vi "Autonomous Independent.vi"() -> ()   [LabVIEW 2016]
doc: "This VI is called when autonomous begins, and will automatically be terminated when autonomous ends. You can carry out timed or sensor driven robot movement independently without needing to return to the caller."
uses:
  <vilib>/Rock Robotics/WPI/Relay/WPI_RelayValue.ctl
  <vilib>/Rock Robotics/WPI/Utilities/WPI_GetSetVariantRefNum.vi
  <vilib>/Rock Robotics/Network Tables/NT Write Numeric Array.vi
  <vilib>/Rock Robotics/Network Tables/NT Read String.vi
  encoder reset.vi
  Encoder Distance.vi
  <vilib>/Rock Robotics/WPI/RobotDrive/WPI_RobotDriveMecanumDrive_Cartesian.vi
  Encoder Rate Shooter.vi
  auto time.vi
  Cam X.vi
panel:
  out "Over Threshold? 3":bool
  out "High Noon (ms) 3":u32
  out "Over 30 Seconds? 3":bool
  out "Over Threshold? 2":bool
  out "High Time (ms) 2":u32
  out "Over 30 Seconds? 2":bool
  in  "Shooter Control 2":dbl
  out "Init Encoder":bool
  out "encoder speed":i32
  # "HIT CONTROL + E"
  # "Be sure to right-click and choose Data Operations>>Make Current Value default if you want to save the array values with the VI"
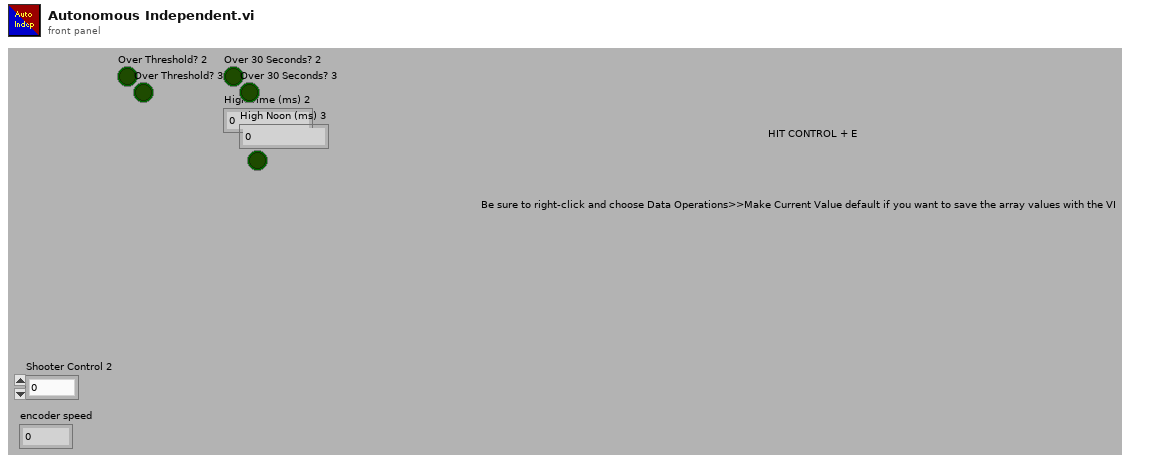
[diagram p1: front panel]
types:
  T1 = typedef "WPI_RelayValue.ctl" = enum16{"Off", "On", "Forward", "Reverse"}
  T2 = typedef "WPI_RelayDevRef.ctl" = cluster{"DevStatus":errorcluster, "Relay Channel":T3, "Relay Direction":T4}
  T3 = typedef "FPGA_DIORelayChannel.ctl" = enum8{"Relay 0", "Relay 1", "Relay 2", "Relay 3", "Invalid"}
  T4 = typedef "WPI_RelayDirection.ctl" = enum16{"Both directions", "Forward only", "Reverse only"}
  T5 = typedef "WPI_JoystickDevRef.ctl" = cluster{"Device":T6}
  T6 = typedef "WPI_JoystickDeviceEnum.ctl" = enum16{"USB 0", "USB 1", "USB 2", "USB 3", "USB 4", "USB 5"}
  T7 = typedef "WPI_RobotDriveDevRef.ctl" = cluster{"DevStatus":errorcluster, "Motors[]":T8[], "Square Inputs":bool, "Max Output":dbl}
  T8 = typedef "WPI_MotorControlDeviceRef.ctl" = cluster{"DeviceStatus":errorcluster, "Type":T9, "PWM":cluster{"PWM Channel":T10, "DeadBand":T11}, "CAN":cluster{"Device Number":u8, "SetOutput VI Ref":variant, "GetOutput VI Ref":variant, "Enable VI Ref":variant, "Disable VI Ref":variant, "Data":variant}, "Invert":bool}
  T9 = typedef "WPI_MotorControlType.ctl" = enum16{"PWM", "CAN"}
  T10 = typedef "FPGA_DIOPWMChannel.ctl" = enum8{"PWM 0", "PWM 1", "PWM 2", "PWM 3", "PWM 4", "PWM 5", "PWM 6", "PWM 7", "PWM 8", "PWM 9", "PWM MXP 0", "PWM MXP 1", "PWM MXP 2", "PWM MXP 3", "PWM MXP 4", "PWM MXP 5", "PWM MXP 6", "PWM MXP 7", "PWM MXP 8", "PWM MXP 9", "Invalid"}
  T11 = typedef "WPI_PWMDeadband.ctl" = cluster{"Name":string, "maxPositivePwm":i32, "minPositivePwm":i32, "centerPwm":i32, "maxNegativePwm":i32, "minNegativePwm":i32, "angularRange":u16}
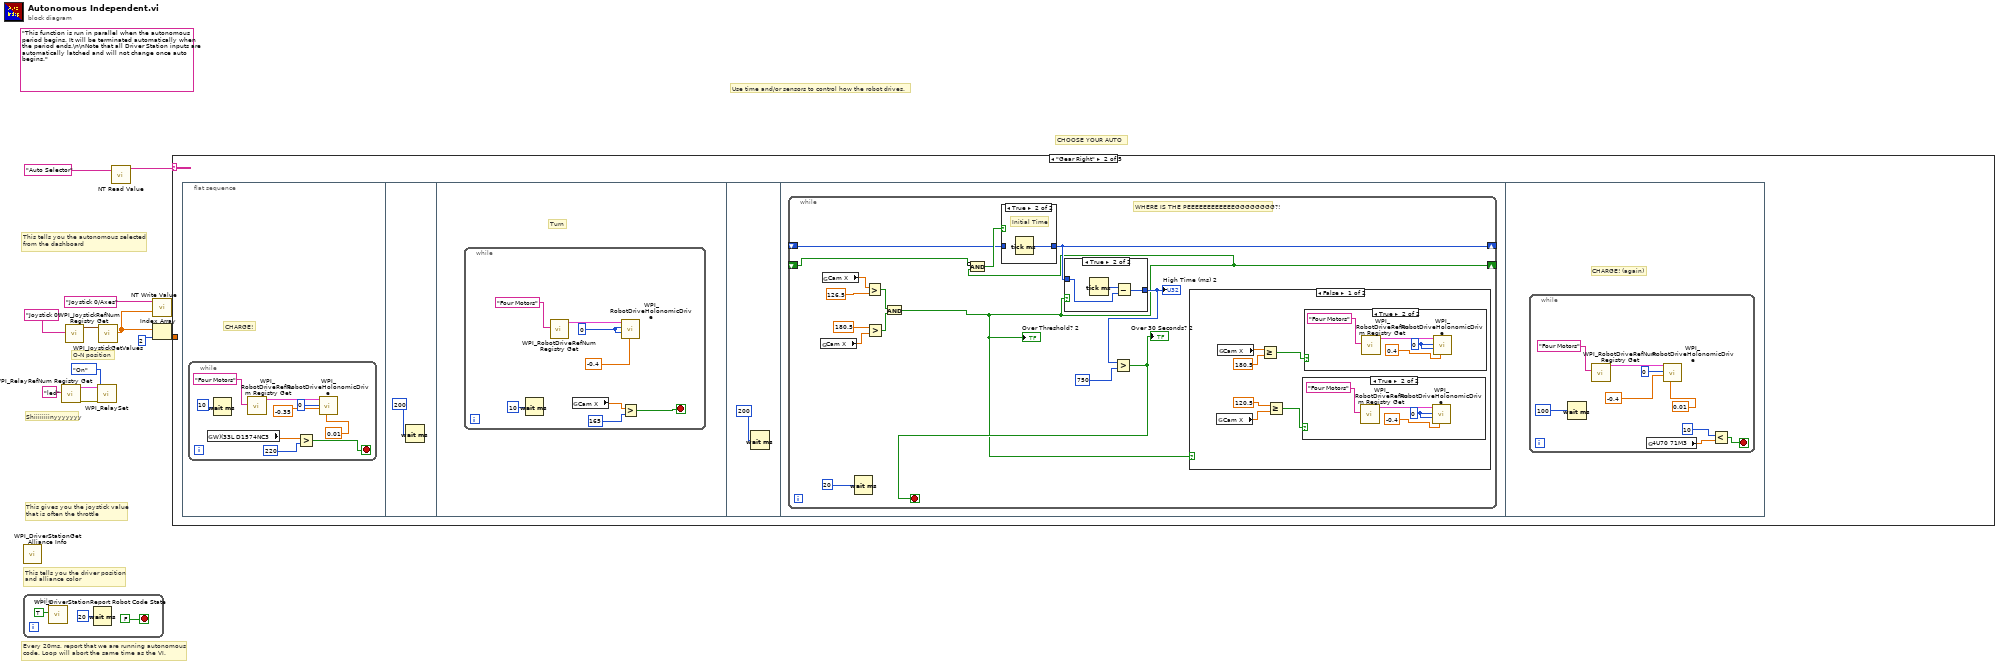
[diagram p0: block diagram]
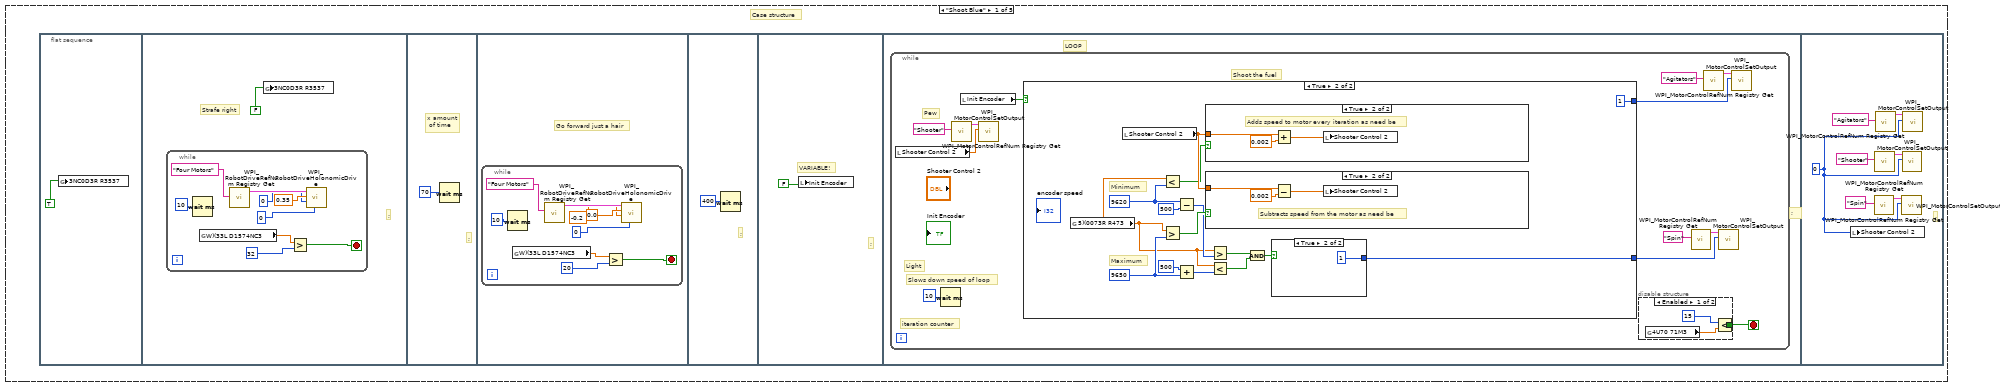
[diagram p2: hidden frame]
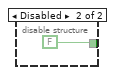
[diagram p3: hidden frame]
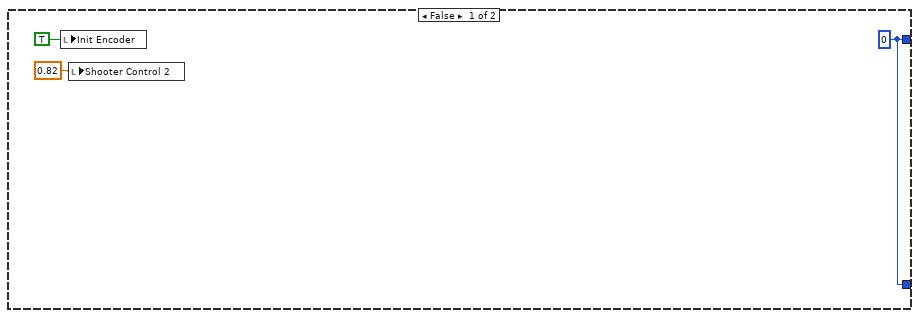
[diagram p4: hidden frame]
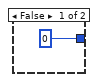
[diagram p5: hidden frame]
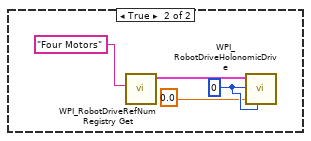
[diagram p10: hidden frame]
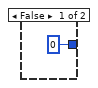
[diagram p11: hidden frame]
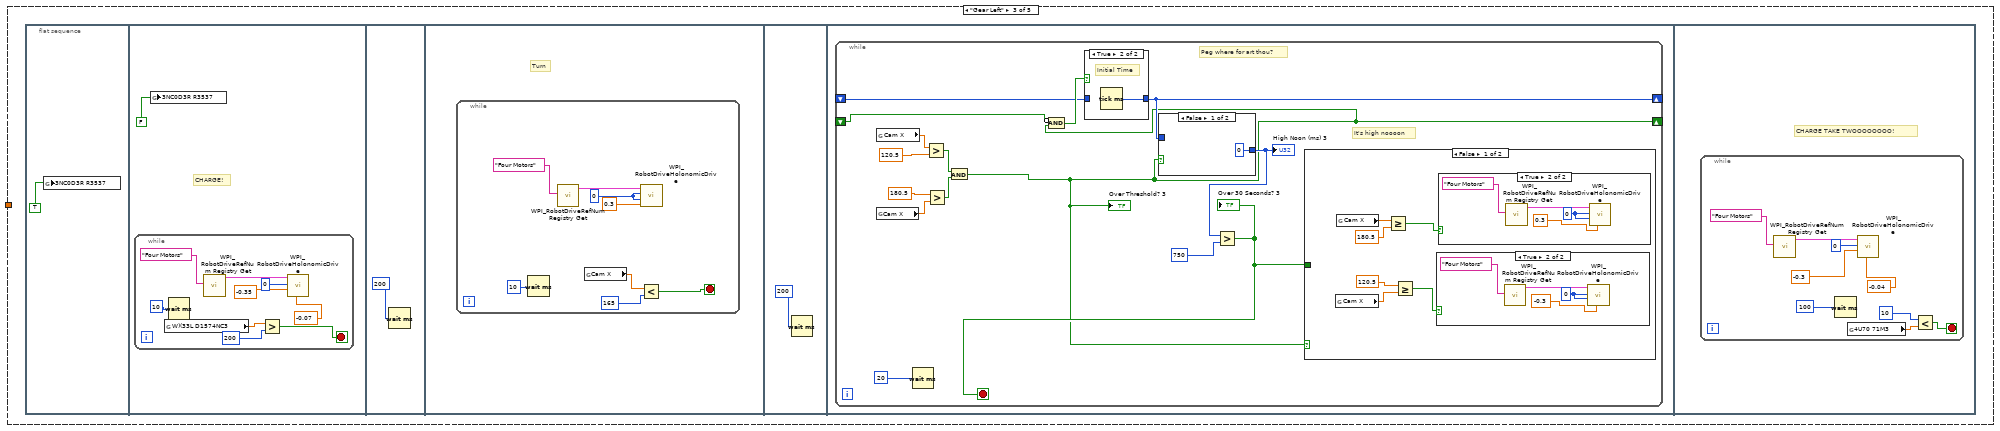
[diagram p13: hidden frame]
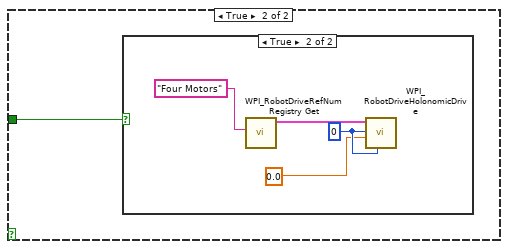
[diagram p16: hidden frame]
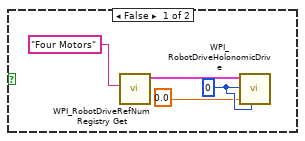
[diagram p17: hidden frame]
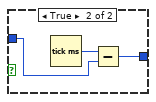
[diagram p18: hidden frame]
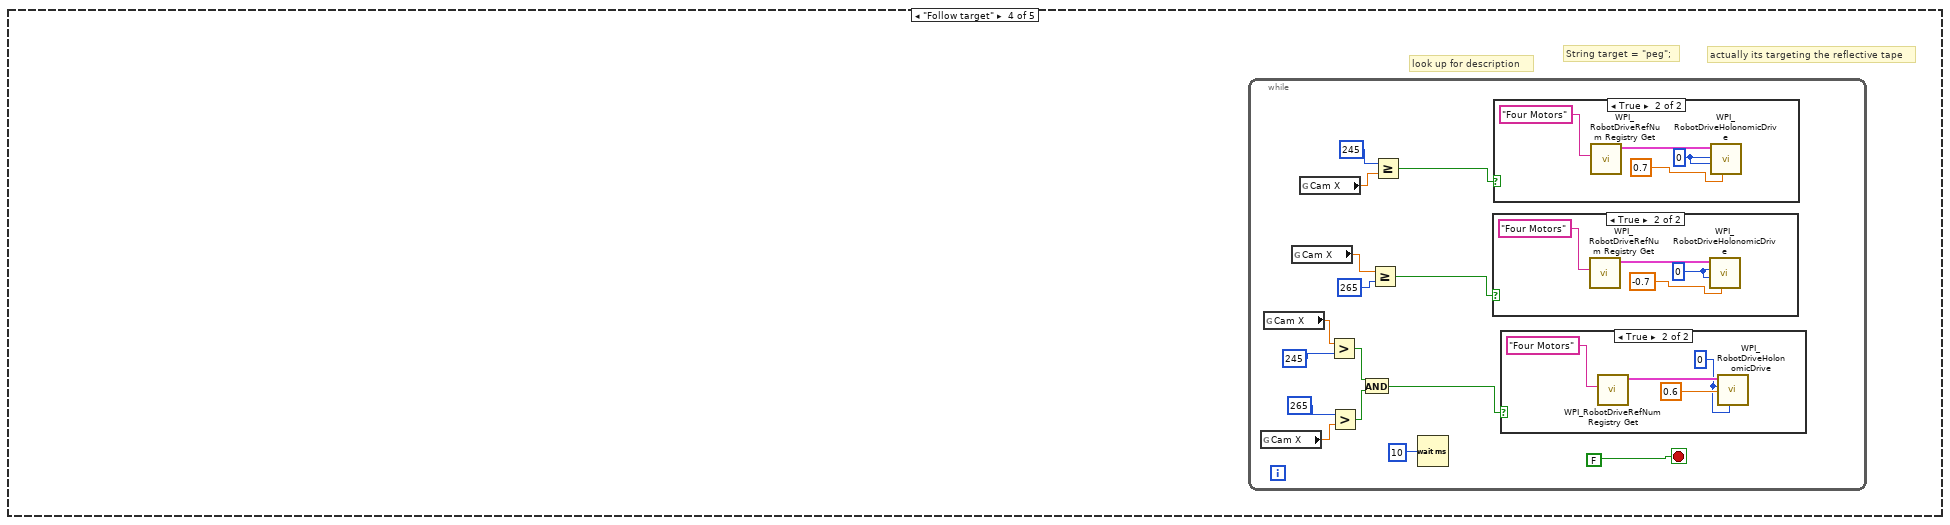
[diagram p20: hidden frame]
diagram:
  (unwired) "This function is run in parallel when the autonomous period begins. It will be terminated automatically when the period ends.\n\nNote that all Driver Station inputs are automatically latched and will not change once auto begins."
  # "Shiiiiiiiinyyyyyyy"
  # "O-N position"
  # "CHOOSE YOUR AUTO"
  # "This tells you the autonomous selected\nfrom the dashboard"
  # "Every 20ms, report that we are running autonomous\ncode. Loop will abort the same time as the VI."
  # "This gives you the joystick value\nthat is often the throttle"
  # "Use time and/or sensors to control how the robot drives."
  # "This tells you the driver position\nand alliance color"
  n1 = call <vilib>:"WPI_DriverStationGet Alliance Info.vi"() -> ()  [unwired: 12 out]
  n2 = while {
    stop <- FALSE stop-if-true
    n3 = call <vilib>:"WPI_DriverStationReport Robot Code State.vi"("Autonomous"=TRUE) -> ()  [unwired: 10 in, 1 out]
    n4 = Wait (ms)(milliseconds to wait=u32 20) -> ()  [unwired: 1 out]
  }
  n5 = call <vilib>:"WPI_RelayRefNum Registry Get.vi"("refnum name"="led") -> ("error out"=w4:errorcluster, "RelayDevRef"=w3:T2)  [unwired: 9 in]
  n6 = call <vilib>:"WPI_JoystickRefNum Registry Get.vi"("refnum name"="Joystick 0") -> ("JoystickDevRef"=w11:T5)  [unwired: 1 in, 9 out]
  n7 = call <vilib>:"WPI_RelaySet.vi"("error in (no error)"=w4, "RelayValue"=WPI_RelayValue."On", "RelayDevRef"=w3) -> ()  [unwired: 7 in, 2 out]
  n8 = call <vilib>:"WPI_JoystickGetValues.vi"("JoystickDevRef"=w11) -> ("Axes"=w7:dbl[])  [unwired: 6 in, 4 out]
  n9 = call-poly <vilib>:"NT Read Value.vi"("Name"="Auto Selector") -> ("String"=w5:string)  [unwired: 9 in, 1 out]
  n10 = call-poly <vilib>:"NT Write Value.vi"("Numeric Array"=w7, "Name"="Joystick 0/Axes") -> ()  [unwired: 9 in, 1 out]
  n11 = Index Array(array=w7, index=u32 2 ("milliseconds to wait")) -> (element=w6:dbl)
  n12 = case shown="\"Gear Right\"" w5 {
    tunnel: w6 -> [_ _ _ _ _]
    frame "Shoot Blue" {
      # "Case structure"
      n13 = flat-sequence {
        frame #0 {
          n14 = global write "encoder reset.vi" "3NC0D3R R3537"(TRUE) -> ()
        }
        frame #1 {
          # "Strafe right"
          # ";"
          n15 = while {
            stop <- w24 stop-if-true
            n16 = Wait (ms)(milliseconds to wait=10) -> ()  [unwired: 1 out]
            n17 = global read "Encoder Distance.vi" "W)(33L D1574NC3"() -> (w18:dbl)
            n18 = call <vilib>:"WPI_RobotDriveRefNum Registry Get.vi"("refnum name"="Four Motors") -> ("RobotDriveDevRef"=w26:T7)  [unwired: 9 in, 1 out]
            n19 = Greater?(x=w18, y=32) -> (0:w24:bool)
            n20 = call-poly <vilib>:"WPI_RobotDriveHolonomicDrive.vi"("Rotation"=0, "Y"=0, "X"=0.35, "RobotDriveDevRef"=w26) -> ()  [unwired: 5 in, 3 out]
          }
          n21 = global write "encoder reset.vi" "3NC0D3R R3537"(FALSE) -> ()
        }
        frame #2 {
          # "x amount\n of time"
          # ";"
          n22 = Wait (ms)(milliseconds to wait=70) -> ()  [unwired: 1 out]
        }
        frame #3 {
          # "Go forward just a hair"
          n23 = while {
            stop <- w34 stop-if-true
            n24 = Wait (ms)(milliseconds to wait=10) -> ()  [unwired: 1 out]
            n25 = global read "Encoder Distance.vi" "W)(33L D1574NC3"() -> (w28:dbl)
            n26 = call <vilib>:"WPI_RobotDriveRefNum Registry Get.vi"("refnum name"="Four Motors") -> ("RobotDriveDevRef"=w36:T7)  [unwired: 9 in, 1 out]
            n27 = Greater?(x=w28, y=20) -> (0:w34:bool)
            n28 = call-poly <vilib>:"WPI_RobotDriveHolonomicDrive.vi"("Rotation"=0, "Y"=-0.2, "X"=0.0, "RobotDriveDevRef"=w36) -> ()  [unwired: 5 in, 3 out]
          }
        }
        frame #4 {
          # ";"
          n29 = Wait (ms)(milliseconds to wait=400) -> ()  [unwired: 1 out]
        }
        frame #5 {
          # "VARIABLE!"
          # ";"
          n30 = local write "Init Encoder"(FALSE) -> ()
        }
        frame #6 {
          # "LOOP"
          # ";"
          n31 = while {
            stop <- w39 stop-if-true
            # "Slows down speed of loop"
            # "Pew"
            # "iteration counter"
            # "Shoot the fuel"
            # "Light"
            n32 = local read "Shooter Control 2"() -> (w40:dbl)
            n33 = Wait (ms)(milliseconds to wait=10) -> ()  [unwired: 1 out]
            n34 = call <vilib>:"WPI_MotorControlRefNum Registry Get.vi"("refnum name"="Shooter") -> ("MotorControlDevRef"=w42:T8)  [unwired: 9 in, 1 out]
            n35 = local read "Init Encoder"() -> (w44:bool)
            n36 = call <vilib>:"WPI_MotorControlSetOutput.vi"("Output"=w40, "MotorControlDevRef"=w42) -> ()  [unwired: 7 in, 3 out]
            n37 = case shown="True" w44 {
              tunnel: [w56 w70] -> w46
              tunnel: [w56 1] -> w45
              frame False {
                w56 = 0
                n38 = local write "Init Encoder"(TRUE) -> ()
                n39 = local write "Shooter Control 2"(0.82) -> ()
              }
              frame True {
                w59 = 9650
                w60 = 9620
                # "Minimum"
                # "Maximum"
                n40 = global read "Encoder Rate Shooter.vi" "5)(0073R R473"() -> (w58:dbl)
                n41 = local read "Shooter Control 2"() -> (w72:dbl)
                n42 = Less?(x=w58, y=w60) -> (x < y?=w69:bool)
                n43 = Greater?(x=w58, y=w59) -> (0:w68:bool)
                n44 = Subtract(x=w60, y=500) -> (x-y=w65:i32)
                n45 = Add(x=500, y=w59) -> (x+y=w64:i32)
                n46 = case shown="True" w69 {
                  tunnel: w72 -> [_ w79]
                  frame False {
                  }
                  frame True {
                    # "Adds speed to motor every iteration as need be"
                    n47 = Add(x=w79, y=0.002) -> (x+y=w78:dbl)
                    n48 = local write "Shooter Control 2"(w78) -> ()
                  }
                }
                n49 = case shown="True" w68 {
                  tunnel: w72 -> [_ w76]
                  frame False {
                  }
                  frame True {
                    # "Subtracts speed from the motor as need be"
                    n50 = Subtract(x=w76, y=0.002) -> (x-y=w75:dbl)
                    n51 = local write "Shooter Control 2"(w75) -> ()
                  }
                }
                n52 = Greater?(x=w58, y=w65) -> (0:w62:bool)
                n53 = Less?(x=w58, y=w64) -> (x < y?=w63:bool)
                n54 = And(x=w62, y=w63) -> (x .and. y?=w71:bool)
                n55 = case shown="True" w71 {
                  tunnel: [0 1] -> w70
                  frame False {
                  }
                  frame True {
                  }
                }
              }
            }
            n56 = disable-structure shown="Enabled" {
              disable-tunnel: [w52 FALSE] -> w39
              frame Enabled {
                n57 = global read "auto time.vi" "4U70 71M3"() -> (w51:dbl)
                n58 = Less?(x=15, y=w51) -> (x < y?=w52:bool)
              }
              frame Disabled {
              }
            }
            n59 = call <vilib>:"WPI_MotorControlRefNum Registry Get.vi"("refnum name"="Spin") -> ("MotorControlDevRef"=w50:T8)  [unwired: 9 in, 1 out]
            n60 = call <vilib>:"WPI_MotorControlRefNum Registry Get.vi"("refnum name"="Agitators") -> ("MotorControlDevRef"=w48:T8)  [unwired: 9 in, 1 out]
            n61 = call <vilib>:"WPI_MotorControlSetOutput.vi"("Output"=w46, "MotorControlDevRef"=w50) -> ()  [unwired: 7 in, 3 out]
            n62 = call <vilib>:"WPI_MotorControlSetOutput.vi"("Output"=w45, "MotorControlDevRef"=w48) -> ()  [unwired: 7 in, 3 out]
          }
        }
        frame #7 {
          w81 = 0
          # ";"
          n63 = local write "Shooter Control 2"(w81) -> ()
          n64 = call <vilib>:"WPI_MotorControlRefNum Registry Get.vi"("refnum name"="Spin") -> ("MotorControlDevRef"=w87:T8)  [unwired: 9 in, 1 out]
          n65 = call <vilib>:"WPI_MotorControlRefNum Registry Get.vi"("refnum name"="Shooter") -> ("MotorControlDevRef"=w83:T8)  [unwired: 9 in, 1 out]
          n66 = call <vilib>:"WPI_MotorControlRefNum Registry Get.vi"("refnum name"="Agitators") -> ("MotorControlDevRef"=w85:T8)  [unwired: 9 in, 1 out]
          n67 = call <vilib>:"WPI_MotorControlSetOutput.vi"("Output"=w81, "MotorControlDevRef"=w87) -> ()  [unwired: 7 in, 3 out]
          n68 = call <vilib>:"WPI_MotorControlSetOutput.vi"("Output"=w81, "MotorControlDevRef"=w83) -> ()  [unwired: 7 in, 3 out]
          n69 = call <vilib>:"WPI_MotorControlSetOutput.vi"("Output"=w81, "MotorControlDevRef"=w85) -> ()  [unwired: 7 in, 3 out]
        }
      }
    }
    frame "Gear Right" {
      n70 = flat-sequence {
        frame #0 {
          # "CHARGE!"
          n71 = while {
            stop <- w93 stop-if-true
            n72 = global read "Encoder Distance.vi" "W)(33L D1574NC3"() -> (w88:dbl)
            n73 = Wait (ms)(milliseconds to wait=10) -> ()  [unwired: 1 out]
            n74 = call <vilib>:"WPI_RobotDriveRefNum Registry Get.vi"("refnum name"="Four Motors") -> ("RobotDriveDevRef"=w96:T7)  [unwired: 9 in, 1 out]
            n75 = Greater?(x=w88, y=220) -> (0:w93:bool)
            n76 = call-poly <vilib>:"WPI_RobotDriveHolonomicDrive.vi"("Rotation"=0.01, "Y"=-0.35, "X"=0, "RobotDriveDevRef"=w96) -> ()  [unwired: 5 in, 3 out]
          }
        }
        frame #1 {
          n77 = Wait (ms)(milliseconds to wait=200) -> ()  [unwired: 1 out]
        }
        frame #2 {
          # "Turn"
          n78 = while {
            stop <- w103 stop-if-true
            w99 = 0
            n79 = Wait (ms)(milliseconds to wait=10) -> ()  [unwired: 1 out]
            n80 = call <vilib>:"WPI_RobotDriveRefNum Registry Get.vi"("refnum name"="Four Motors") -> ("RobotDriveDevRef"=w102:T7)  [unwired: 9 in, 1 out]
            n81 = global read "Cam X.vi" "Cam X"() -> (w98:dbl)
            n82 = call-poly <vilib>:"WPI_RobotDriveHolonomicDrive.vi"("Rotation"=-0.4, "Y"=w99, "X"=w99, "RobotDriveDevRef"=w102) -> ()  [unwired: 5 in, 3 out]
            n83 = Greater?(x=w98, y=165) -> (0:w103:bool)
          }
        }
        frame #3 {
          n84 = Wait (ms)(milliseconds to wait=200) -> ()  [unwired: 1 out]
        }
        frame #4 {
          n85 = while {
            shift-right: [w119] -> _
            shift-left: _ -> [w120]
            shift-right: [w109] -> _
            shift-left: _ -> [w118]
            stop <- w112 stop-if-true
            # "WHERE IS THE PEEEEEEEEEEEEGGGGGGGG?!"
            n86 = global read "Cam X.vi" "Cam X"() -> (w107:dbl)
            n87 = global read "Cam X.vi" "Cam X"() -> (w108:dbl)
            n88 = Wait (ms)(milliseconds to wait=20) -> ()  [unwired: 1 out]
            n89 = Greater?(x=w108, y=126.5) -> (0:w116:bool)
            n90 = Greater?(x=180.5, y=w107) -> (0:w117:bool)
            n91 = And(x=w116, y=w117) -> (x .and. y?=w109:bool)
            "Over Threshold? 2" <- w109
            n92 = Compound Arithmetic op=AND(invert w118, w109) -> (w121:bool)
            n93 = case shown="True" w121 {
              tunnel: [w144 w145] -> w119
              tunnel: w120 -> [w144 _]
              frame False {
              }
              frame True {
                # "Initial Time"
                n94 = Tick Count (ms)() -> (millisecond timer value=w145:u32)
              }
            }
            n95 = case shown="True" w109 {
              tunnel: w119 -> [_ w142]
              tunnel: [u32 0 w141] -> w111
              frame False {
              }
              frame True {
                n96 = Tick Count (ms)() -> (millisecond timer value=w143:u32)
                n97 = Subtract(x=w143, y=w142) -> (x-y=w141:u32)
              }
            }
            "High Time (ms) 2" <- w111
            n98 = Greater?(x=w111, y=u32 750) -> (0:w112:bool)
            "Over 30 Seconds? 2" <- w112
            n99 = case shown="False" w109 {
              frame False {
                n100 = global read "Cam X.vi" "Cam X"() -> (w125:dbl)
                n101 = global read "Cam X.vi" "Cam X"() -> (w127:dbl)
                n102 = Greater Or Equal?(x=w127, y=180.5) -> (x >= y?=w122:bool)
                n103 = Greater Or Equal?(x=120.5, y=w125) -> (x >= y?=w123:bool)
                n104 = case shown="True" w123 {
                  frame False {
                  }
                  frame True {
                    w128 = 0
                    n105 = call <vilib>:"WPI_RobotDriveRefNum Registry Get.vi"("refnum name"="Four Motors") -> ("RobotDriveDevRef"=w131:T7)  [unwired: 9 in, 1 out]
                    n106 = call-poly <vilib>:"WPI_RobotDriveHolonomicDrive.vi"("Rotation"=-0.4, "Y"=w128, "X"=w128, "RobotDriveDevRef"=w131) -> ()  [unwired: 5 in, 3 out]
                  }
                }
                n107 = case shown="True" w122 {
                  frame False {
                  }
                  frame True {
                    w132 = 0
                    n108 = call <vilib>:"WPI_RobotDriveRefNum Registry Get.vi"("refnum name"="Four Motors") -> ("RobotDriveDevRef"=w135:T7)  [unwired: 9 in, 1 out]
                    n109 = call-poly <vilib>:"WPI_RobotDriveHolonomicDrive.vi"("Rotation"=0.4, "Y"=w132, "X"=w132, "RobotDriveDevRef"=w135) -> ()  [unwired: 5 in, 3 out]
                  }
                }
              }
              frame True {
                w137 = 0
                n110 = call <vilib>:"WPI_RobotDriveRefNum Registry Get.vi"("refnum name"="Four Motors") -> ("RobotDriveDevRef"=w139:T7)  [unwired: 9 in, 1 out]
                n111 = call-poly <vilib>:"WPI_RobotDriveHolonomicDrive.vi"("Rotation"=w137, "Y"=0.0, "X"=w137, "RobotDriveDevRef"=w139) -> ()  [unwired: 5 in, 3 out]
              }
            }
          }
        }
        frame #5 {
          # "CHARGE! (again)"
          n112 = while {
            stop <- w148 stop-if-true
            n113 = Wait (ms)(milliseconds to wait=100) -> ()  [unwired: 1 out]
            n114 = call <vilib>:"WPI_RobotDriveRefNum Registry Get.vi"("refnum name"="Four Motors") -> ("RobotDriveDevRef"=w154:T7)  [unwired: 9 in, 1 out]
            n115 = global read "auto time.vi" "4U70 71M3"() -> (w146:dbl)
            n116 = call-poly <vilib>:"WPI_RobotDriveHolonomicDrive.vi"("Rotation"=0.01, "Y"=-0.4, "X"=0, "RobotDriveDevRef"=w154) -> ()  [unwired: 5 in, 3 out]
            n117 = Less?(x=10, y=w146) -> (x < y?=w148:bool)
          }
        }
      }
    }
    frame "Gear Left" {
      n118 = flat-sequence {
        frame #0 {
          n119 = global write "encoder reset.vi" "3NC0D3R R3537"(TRUE) -> ()
        }
        frame #1 {
          # "CHARGE!"
          n120 = while {
            stop <- w162 stop-if-true
            n121 = global read "Encoder Distance.vi" "W)(33L D1574NC3"() -> (w157:dbl)
            n122 = Wait (ms)(milliseconds to wait=10) -> ()  [unwired: 1 out]
            n123 = call <vilib>:"WPI_RobotDriveRefNum Registry Get.vi"("refnum name"="Four Motors") -> ("RobotDriveDevRef"=w165:T7)  [unwired: 9 in, 1 out]
            n124 = Greater?(x=w157, y=200) -> (0:w162:bool)
            n125 = call-poly <vilib>:"WPI_RobotDriveHolonomicDrive.vi"("Rotation"=-0.07, "Y"=-0.35, "X"=0, "RobotDriveDevRef"=w165) -> ()  [unwired: 5 in, 3 out]
          }
          n126 = global write "encoder reset.vi" "3NC0D3R R3537"(FALSE) -> ()
        }
        frame #2 {
          n127 = Wait (ms)(milliseconds to wait=200) -> ()  [unwired: 1 out]
        }
        frame #3 {
          # "Turn"
          n128 = while {
            stop <- w172 stop-if-true
            w167 = 0
            n129 = Wait (ms)(milliseconds to wait=10) -> ()  [unwired: 1 out]
            n130 = call <vilib>:"WPI_RobotDriveRefNum Registry Get.vi"("refnum name"="Four Motors") -> ("RobotDriveDevRef"=w171:T7)  [unwired: 9 in, 1 out]
            n131 = global read "Cam X.vi" "Cam X"() -> (w169:dbl)
            n132 = call-poly <vilib>:"WPI_RobotDriveHolonomicDrive.vi"("Rotation"=0.3, "Y"=w167, "X"=w167, "RobotDriveDevRef"=w171) -> ()  [unwired: 5 in, 3 out]
            n133 = Less?(x=w169, y=165) -> (x < y?=w172:bool)
          }
        }
        frame #4 {
          n134 = Wait (ms)(milliseconds to wait=200) -> ()  [unwired: 1 out]
        }
        frame #5 {
          n135 = while {
            shift-right: [w188] -> _
            shift-left: _ -> [w189]
            shift-right: [w176] -> _
            shift-left: _ -> [w187]
            stop <- w179 stop-if-true
            # "It's high noooon"
            # "Peg where for art thou?"
            n136 = global read "Cam X.vi" "Cam X"() -> (w185:dbl)
            n137 = global read "Cam X.vi" "Cam X"() -> (w186:dbl)
            n138 = Wait (ms)(milliseconds to wait=20) -> ()  [unwired: 1 out]
            n139 = Greater?(x=w186, y=120.5) -> (0:w183:bool)
            n140 = Greater?(x=180.5, y=w185) -> (0:w184:bool)
            n141 = And(x=w183, y=w184) -> (x .and. y?=w176:bool)
            "Over Threshold? 3" <- w176
            n142 = Compound Arithmetic op=AND(invert w187, w176) -> (w190:bool)
            n143 = case shown="True" w190 {
              tunnel: [w218 w219] -> w188
              tunnel: w189 -> [w218 _]
              frame False {
              }
              frame True {
                # "Initial Time"
                n144 = Tick Count (ms)() -> (millisecond timer value=w219:u32)
              }
            }
            n145 = case shown="False" w176 {
              tunnel: w188 -> [_ w216]
              tunnel: [u32 0 w215] -> w178
              frame False {
              }
              frame True {
                n146 = Tick Count (ms)() -> (millisecond timer value=w217:u32)
                n147 = Subtract(x=w217, y=w216) -> (x-y=w215:u32)
              }
            }
            "High Noon (ms) 3" <- w178
            n148 = Greater?(x=w178, y=u32 750) -> (0:w179:bool)
            "Over 30 Seconds? 3" <- w179
            n149 = case shown="False" w176 {
              tunnel: w179 -> [_ w205]
              frame False {
                n150 = global read "Cam X.vi" "Cam X"() -> (w194:dbl)
                n151 = global read "Cam X.vi" "Cam X"() -> (w196:dbl)
                n152 = Greater Or Equal?(x=w196, y=180.5) -> (x >= y?=w191:bool)
                n153 = Greater Or Equal?(x=120.5, y=w194) -> (x >= y?=w192:bool)
                n154 = case shown="True" w192 {
                  frame False {
                  }
                  frame True {
                    w197 = 0
                    n155 = call <vilib>:"WPI_RobotDriveRefNum Registry Get.vi"("refnum name"="Four Motors") -> ("RobotDriveDevRef"=w200:T7)  [unwired: 9 in, 1 out]
                    n156 = call-poly <vilib>:"WPI_RobotDriveHolonomicDrive.vi"("Rotation"=-0.3, "Y"=w197, "X"=w197, "RobotDriveDevRef"=w200) -> ()  [unwired: 5 in, 3 out]
                  }
                }
                n157 = case shown="True" w191 {
                  frame False {
                  }
                  frame True {
                    w201 = 0
                    n158 = call <vilib>:"WPI_RobotDriveRefNum Registry Get.vi"("refnum name"="Four Motors") -> ("RobotDriveDevRef"=w204:T7)  [unwired: 9 in, 1 out]
                    n159 = call-poly <vilib>:"WPI_RobotDriveHolonomicDrive.vi"("Rotation"=0.3, "Y"=w201, "X"=w201, "RobotDriveDevRef"=w204) -> ()  [unwired: 5 in, 3 out]
                  }
                }
              }
              frame True {
                n160 = case shown="True" w205 {
                  frame False {
                    w207 = 0
                    n161 = call <vilib>:"WPI_RobotDriveRefNum Registry Get.vi"("refnum name"="Four Motors") -> ("RobotDriveDevRef"=w209:T7)  [unwired: 9 in, 1 out]
                    n162 = call-poly <vilib>:"WPI_RobotDriveHolonomicDrive.vi"("Rotation"=w207, "Y"=0.0, "X"=w207, "RobotDriveDevRef"=w209) -> ()  [unwired: 5 in, 3 out]
                  }
                  frame True {
                    w211 = 0
                    n163 = call <vilib>:"WPI_RobotDriveRefNum Registry Get.vi"("refnum name"="Four Motors") -> ("RobotDriveDevRef"=w213:T7)  [unwired: 9 in, 1 out]
                    n164 = call-poly <vilib>:"WPI_RobotDriveHolonomicDrive.vi"("Rotation"=w211, "Y"=0.0, "X"=w211, "RobotDriveDevRef"=w213) -> ()  [unwired: 5 in, 3 out]
                  }
                }
              }
            }
          }
        }
        frame #6 {
          # "CHARGE TAKE TWOOOOOOOO!"
          n165 = while {
            stop <- w222 stop-if-true
            n166 = call <vilib>:"WPI_RobotDriveRefNum Registry Get.vi"("refnum name"="Four Motors") -> ("RobotDriveDevRef"=w228:T7)  [unwired: 9 in, 1 out]
            n167 = Wait (ms)(milliseconds to wait=100) -> ()  [unwired: 1 out]
            n168 = global read "auto time.vi" "4U70 71M3"() -> (w220:dbl)
            n169 = call-poly <vilib>:"WPI_RobotDriveHolonomicDrive.vi"("Rotation"=-0.04, "Y"=-0.3, "X"=0, "RobotDriveDevRef"=w228) -> ()  [unwired: 5 in, 3 out]
            n170 = Less?(x=10, y=w220) -> (x < y?=w222:bool)
          }
        }
      }
    }
    frame "Follow target" {
      # "actually its targeting the reflective tape"
      # "String target = \"peg\";"
      # "look up for description"
      n171 = while {
        stop <- FALSE stop-if-true
        n172 = global read "Cam X.vi" "Cam X"() -> (w233:dbl)
        n173 = global read "Cam X.vi" "Cam X"() -> (w234:dbl)
        n174 = global read "Cam X.vi" "Cam X"() -> (w235:dbl)
        n175 = global read "Cam X.vi" "Cam X"() -> (w236:dbl)
        n176 = Greater?(x=w234, y=245) -> (0:w238:bool)
        n177 = Greater?(x=265, y=w233) -> (0:w237:bool)
        n178 = And(x=w238, y=w237) -> (x .and. y?=w229:bool)
        n179 = Greater Or Equal?(x=w235, y=265) -> (x >= y?=w230:bool)
        n180 = Greater Or Equal?(x=245, y=w236) -> (x >= y?=w231:bool)
        n181 = Wait (ms)(milliseconds to wait=10) -> ()  [unwired: 1 out]
        n182 = case shown="True" w230 {
          frame False {
          }
          frame True {
            w248 = 0
            n183 = call <vilib>:"WPI_RobotDriveRefNum Registry Get.vi"("refnum name"="Four Motors") -> ("RobotDriveDevRef"=w251:T7)  [unwired: 9 in, 1 out]
            n184 = call-poly <vilib>:"WPI_RobotDriveHolonomicDrive.vi"("Rotation"=-0.7, "Y"=w248, "X"=w248, "RobotDriveDevRef"=w251) -> ()  [unwired: 5 in, 3 out]
          }
        }
        n185 = case shown="True" w231 {
          frame False {
          }
          frame True {
            w252 = 0
            n186 = call <vilib>:"WPI_RobotDriveRefNum Registry Get.vi"("refnum name"="Four Motors") -> ("RobotDriveDevRef"=w255:T7)  [unwired: 9 in, 1 out]
            n187 = call-poly <vilib>:"WPI_RobotDriveHolonomicDrive.vi"("Rotation"=0.7, "Y"=w252, "X"=w252, "RobotDriveDevRef"=w255) -> ()  [unwired: 5 in, 3 out]
          }
        }
        n188 = case shown="True" w229 {
          frame False {
          }
          frame True {
            w244 = 0
            n189 = call <vilib>:"WPI_RobotDriveRefNum Registry Get.vi"("refnum name"="Four Motors") -> ("RobotDriveDevRef"=w247:T7)  [unwired: 9 in, 1 out]
            n190 = call-poly <vilib>:"WPI_RobotDriveHolonomicDrive.vi"("Rotation"=w244, "Y"=0.6, "X"=w244, "RobotDriveDevRef"=w247) -> ()  [unwired: 5 in, 3 out]
          }
        }
      }
    }
    frame "Center Gear", Default {
      n191 = while {
        stop <- w256 stop-if-true
        n192 = Wait (ms)(milliseconds to wait=10) -> ()  [unwired: 1 out]
        n193 = global read "auto time.vi" "4U70 71M3"() -> (w257:dbl)
        n194 = call <vilib>:"WPI_RobotDriveRefNum Registry Get.vi"("refnum name"="Four Motors") -> ("RobotDriveDevRef"=w264:T7)  [unwired: 9 in, 1 out]
        n195 = Less?(x=10, y=w257) -> (x < y?=w256:bool)
        n196 = call-poly <vilib>:"WPI_RobotDriveHolonomicDrive.vi"("Rotation"=-0.07, "Y"=-0.35, "X"=0, "RobotDriveDevRef"=w264) -> ()  [unwired: 5 in, 3 out]
      }
    }
  }
